vi "Query Status Register.vi"(8 "error in":errorcluster, 11 "69X_79X in":refnum<class "69X_79X.lvclass">) -> (0 "error out":errorcluster, 3 "69X_79X out":refnum<class "69X_79X.lvclass">)   [LabVIEW 2019, in "69X_79X.lvlib" / "69X_79X.lvclass"]
doc: "Child classes must override this VI:\n\nThis VI is the device specific query of the supply's status registers. \nThe return values are: \n\nThe implementation must read status registers and push the status register values to private data for:\nOCP Flag, OVP Flag, Interlock Flag, Output Flag into the private data arrays of the power supply class."
uses:
  Library/69X_79X.lvclass
  C:/Users/Public/Documents/Development/builds/Instruments/PowerSupply.lvlibp/Library/PowerSupply.lvclass
  builds/Instruments/PowerSupply.lvlibp/Custom Controls/Status_Flags.ctl
  Library/69X_79X.lvclass/69X_79X.ctl
  builds/Instruments/PowerSupply.lvlibp/Accessors/Write Status Flags.vi
  <instrlib>/Agilent N6900 N7900 Series/Agilent N6900 N7900 Series.lvlib
  builds/Instruments/PowerSupply.lvlibp/Library/PowerSupply.lvclass
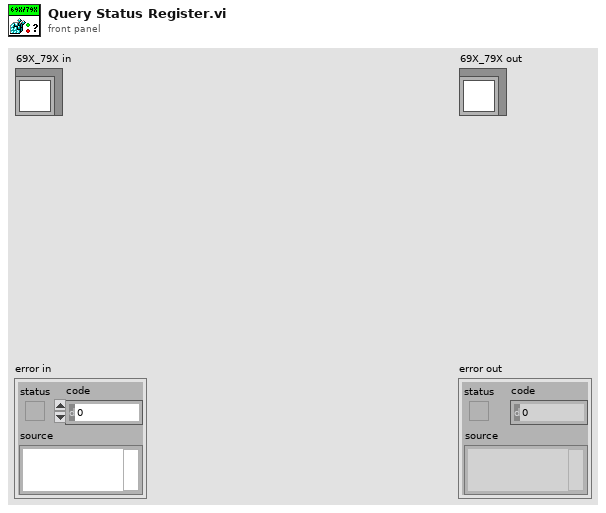
[diagram p1: front panel]
types:
  T1 = typedef "PowerSupply.lvlibp/PowerSupply.lvclass/Status_Flags.ctl" = cluster{"Interlock":bool, "OVP":bool, "OCP":bool, "Output":bool}
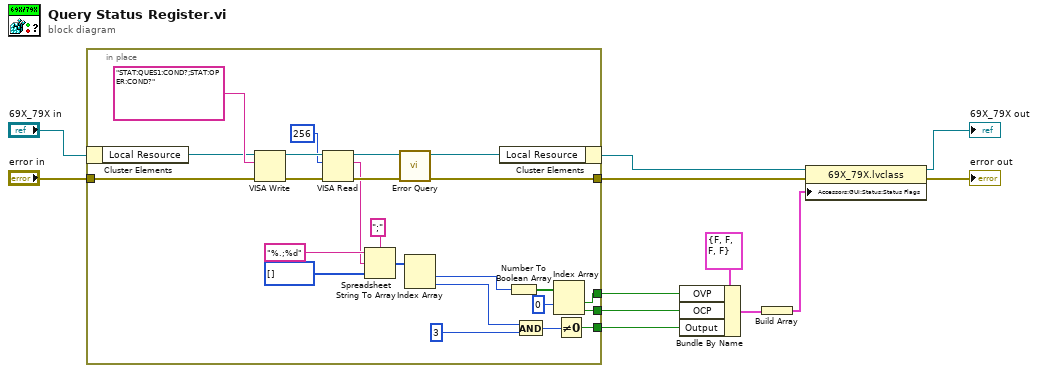
[diagram p0: block diagram]
diagram:
  n1 = in-place {
    in-place-border: "error in" -> [w28]
    in-place-border: [w27] -> w6
    in-place-border: [w17] -> w10
    in-place-border: [w14] -> w8
    in-place-border: [w13] -> w9
    n2 = in-place-cluster #1("69X_79X in") -> ("Local Resource"=w31:refnum<visa-resource-name>)
    n3 = VISA Write(VISA resource name=w31, write buffer="STAT:QUES1:COND?;STAT:OPER:COND?", error in (no error)=w28) -> (VISA resource name out=w34:refnum<visa-resource-name>, error out=w33:errorcluster)  [unwired: 1 out]
    n4 = VISA Read(VISA resource name=w34, byte count=u32 256, error in (no error)=w33) -> (VISA resource name out=w35:refnum<visa-resource-name>, read buffer=w23:string, error out=w36:errorcluster)  [unwired: 1 out]
    n5 = Spreadsheet String To Array(delimiter (Tab)=";", format string="%.;%d", spreadsheet string=w23, array type (2D Dbl)=u32[] []) -> (array=w22:u32[])
    n6 = call <instrlib>:"Error Query.vi"("error in (no error)"=w36, "VISA resource name"=w35) -> ("error out"=w27:errorcluster, "VISA resource name out"=w30:refnum<visa-resource-name>)  [unwired: 6 in, 2 out]
    n7 = Index Array(array=w22) -> (element #1=w21:u32, element #2=w20:u32)  [unwired: 2 in]
    n8 = in-place-cluster #1("Local Resource"=w30) -> (w5:refnum<class "69X_79X.lvclass">)
    n9 = Number To Boolean Array(number=w21) -> (Boolean array=w16:bool[])
    n10 = And(x=w20, y=u32 3 ("x")) -> (x .and. y?=w18:u32)
    n11 = Index Array(array=w16, index #1=0 ("index")) -> (element #1=w14:bool, element #2=w13:bool)  [unwired: 1 in]
    n12 = Not Equal To 0?(x=w18) -> (x != 0?=w17:bool)
  }
  n13 = Bundle By Name(cluster=T1 {"Interlock"=FALSE, "OVP"=FALSE, "OCP"=FALSE, "Output"=FALSE} ("Status"), "OVP"=w8, "OCP"=w9, "Output"=w10) -> (w11:T1)
  n14 = Build Array(w11) -> (w12:T1[])
  n15 = property class="69X_79X.lvclass"(reference=w5, error in=w6, "Accessors:GUI:Status:Status Flags"=w12) -> (reference out=→"69X_79X out":refnum<class "69X_79X.lvclass">, error out=→"error out":errorcluster)
